vi "Vision-dynamic-pump.vi"() -> ()   [LabVIEW 2013]
doc: "Use this template to build a standard state machine design pattern. Each state executes code and determines which state to transition to. Contrast this design pattern with the User Interface Event Handler pattern, in which code executes in response to user actions. Contrast this design pattern also with the Queued Message Handler pattern, in which each message handling code can queue zero or more new messages."
uses:
  StateMachineStates 1.ctl
  <vilib>/DAQmx/read.llb/DAQmx Read (Counter DBL 1Chan 1Samp).vi
  <vilib>/DAQmx/create/channels.llb/DAQmx Create Channel (CI-Pulse Width).vi
  <vilib>/DAQmx/miscellaneous.llb/DAQmx Fill In Error Info.vi
panel:
  in  "Entrainment":bool=TRUE
  in  "Sound at \nstimulus end":bool
  in  "Manual \nvoltage (V)":dbl=2.6 format="%.2p"
  in  "Manual \nphoton #":i64=100
  out "L/R WP target":dbl
  out "List of axes":i32[](array[numeric])
  out "List of WP errors":bool[](array[boolean])
  out "WP error":bool
  out "appended array":dbl[][](array[numeric])
  out "Pump WP":dbl format="%.2f"
  in  "Trigger rate at \n52.6 degrees":dbl=2646.0 format="%.2p"
  in  "Target trial \nlength (ms)":dbl=500.0 format="%.2p"
  in  "Default pump \nWP angle":dbl=52.6
  in  "Pump WP":bool=TRUE
  out "Photon time (ms)":dbl format="%.2f"
  in  "Interval (ms)":u32
  out "Repetition":dbl
  in  "Repetitions":dbl=1.0
  out "WP time (ms)":u32
  out "VISA Handle out":refnum<visa-resource-name>="ASRL5::INSTR"
  out "Initializing":bool
  out "Trial mode":enum16{"Single Photons", "LED", "Mixed LED"}(ring)
  in  "Frequency of LED trials\nfor Mixed mode":dbl=30.0
  out "Bright trial\nrequested":bool
  out "Observer Ready":bool
  in  "Bright/mixed mode \nLED voltage (V)":dbl=2.6 min=-3.0 max=4.0 format="%.2f"
  in  "GPIB address":string="15"
  in  "Period (ms)":i64=20
  in  "Pulse \nlength (ms)":dbl=50.0
  out "L/R WP":dbl format="%.2f"
  in  "Manually \ninitialize":bool
  in  "COM for WPs":u8=3
  out "Blocked trial #":i32
  out "Photon #":i32
  out "LED Voltage":dbl
  in  "Blocking requirements":cluster{"Value":dbl, " Number":i32}[](array[cluster])
  in  "Manual":bool
  in  "Path":path=path "C:/Users/Lab/Dropbox/Vision software/Data"
  out "Counts 2":u32
  out "Counts 1":u32
  in  "Delay for APDs (ms)":u32=25
  in  "Counter 2":tag="Dev1/ctr1"
  in  "Counter 1":tag="Dev1/ctr0"
  out "Trial #":i32
  in  "Mode":enum16{"Single Photons", "LED", "Mixed"}(ring)=enum."Mixed"
  in  "Audio":bool=TRUE
  in  "Self-paced":bool
  out "Stimulus":bool
  out "Location Set":bool
  out "Stimulus \nlocation":string
  out "Waiting":bool
  out "Observer Responded":bool
  out "Response \ntime (ms)":dbl
  out "Observer \nchoice":string
  out "Confidence":i32
  in  "stop":bool
  in  "Next Trial":bool
  in  "Create New File":bool
  out "Subject #":string
  # "Settings for Blocking\nand Mixed Mode"
  # "Instructions: Run VI. Enter blocking requirements, then press\nCreate New File. Initialize waveplates if necessary, and set\nhighlighted controls to desired values. Press Next Trial to begin."
  # "Researcher Interface"
  # "Trial Options"
  # "Counter Options"
  # "Trial Information"
  # "(1)"
  # "(3)"
  # "LED Options"
  # "Pump Settings"
  # "Troubleshooting"
  # "Waveplates"
  # "(2)"
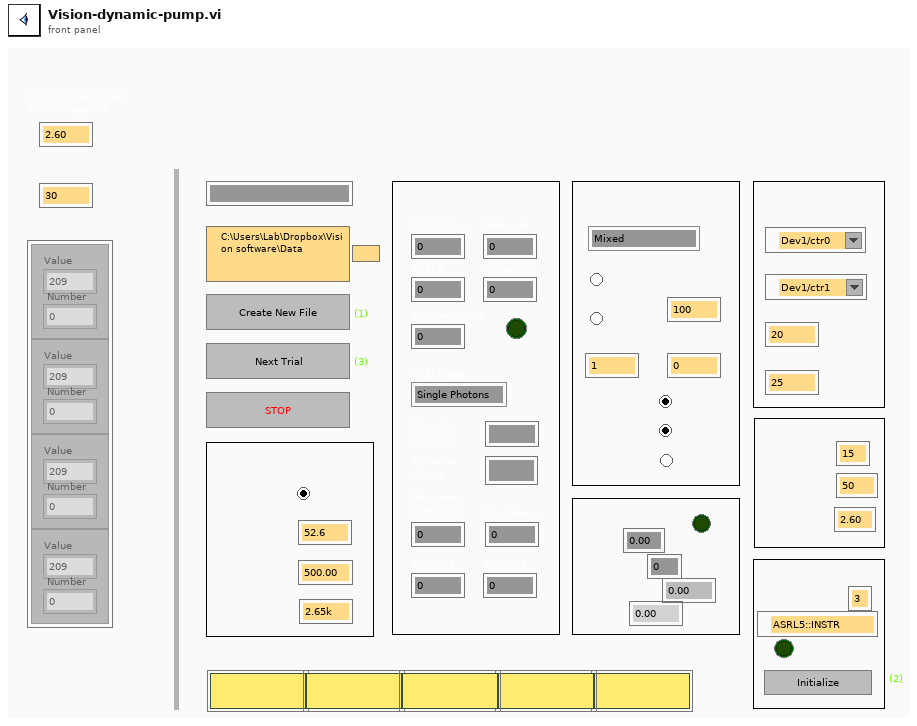
[diagram p1: front panel]
types:
  T1 = typedef "StateMachineStates 1.ctl" = enum16{"WaitResearcher", "Setup", "SetWP", "WaveplateError", "WaitObserverReady", "Photons", "LED", "WaitObserverResponse", "CleanUp", "Stop"}
  T2 = enum16{"0", "1", "2", "3", "4", "5", "6", "7", "8", "9", "A", "B", "C", "D", "E", "F", "G", "H", "I", "J", "K", "L", "M", "N", "O", "P", "Q", "R", "S", "T", "U", "V", "W", "X", "Y", "Z", "F1", "F2", "F3", "F4", "F5", "F6", "F7", "F8", "F9", "F10", "F11", "F12", "F13", "F14", "F15", "ADD", "BACK", "BACKSLASH", "CAPITAL", "COMMA", "DECIMAL", "DELETE", "DIVIDE", "DOWN", "END", "EQUALS", "ESCAPE", "GRAVE (`)", "HOME", "INSERT", "LBRACKET", "LCONTROL", "LEFT", "L ALT", "LSHIFT", "LWIN", "MINUS", "MULTIPLY", "NEXT", "NUMLOCK", "NUMPAD_0", "NUMPAD_1", "NUMPAD_2", "NUMPAD_3", "NUMPAD_4", "NUMPAD_5", "NUMPAD_6", "NUMPAD_7", "NUMPAD_8", "NUMPAD_9", "PAUSE", "PERIOD", "PRIOR (PG UP)", "RBRACKET", "RCONTROL", "RETURN", "RIGHT", "R ALT", "RSHIFT", "RWIN", "SCROLL", "SEMICOLON", "SLASH", "SPACE", "SUBTRACT", "TAB", "UP", "ENTER (num pad)", "' (quote)"}
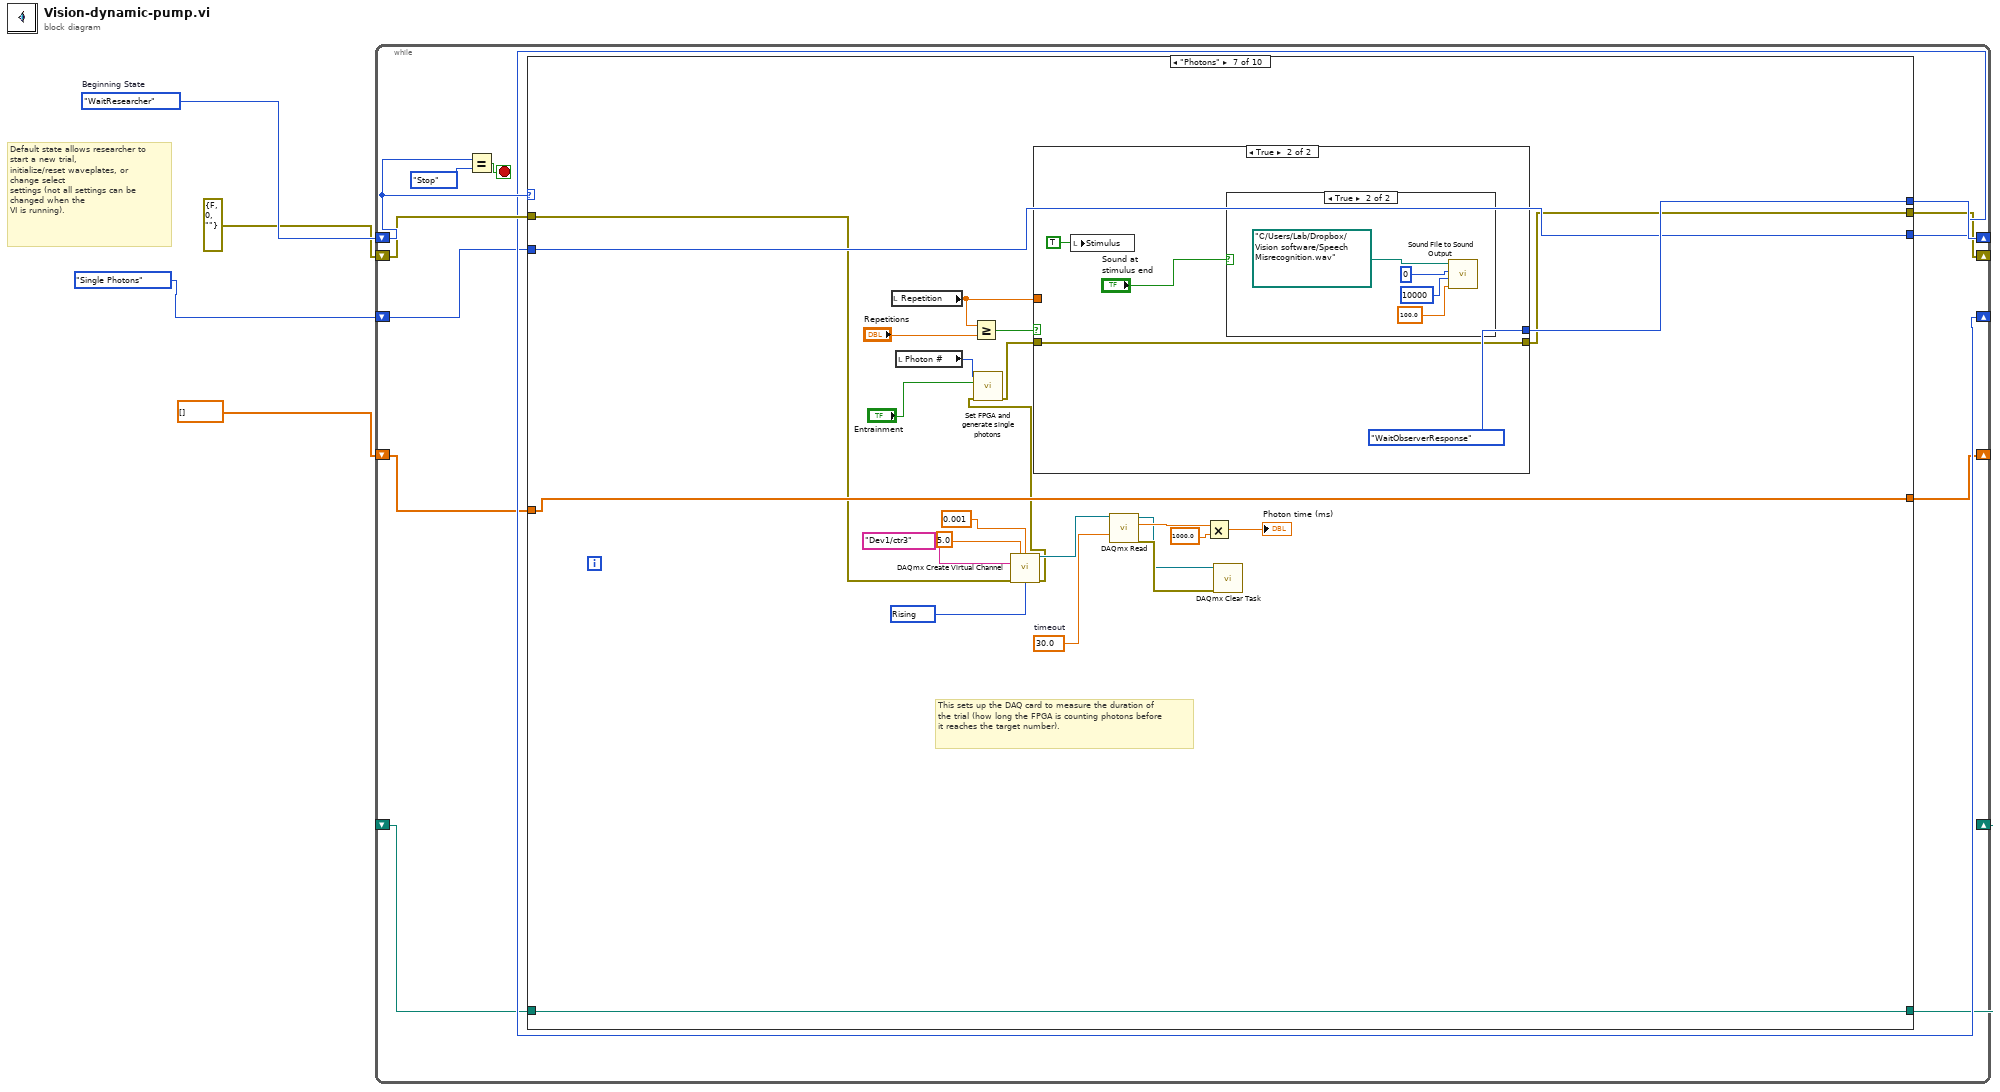
[diagram p0: block diagram]
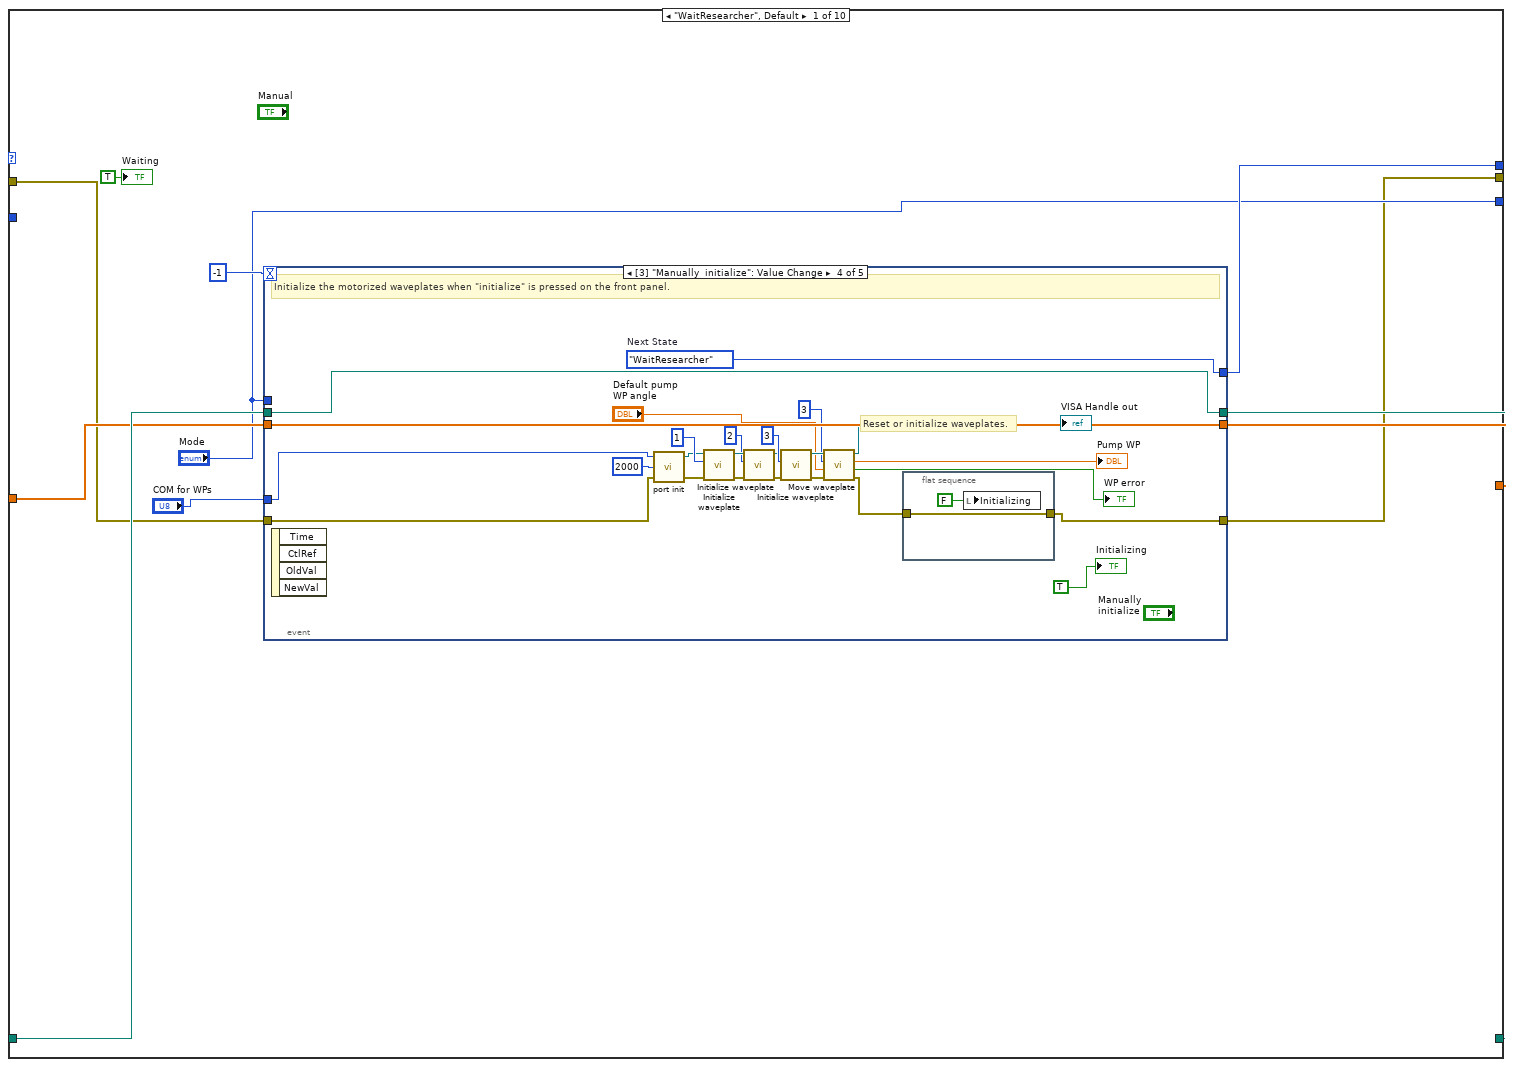
[diagram p2: hidden frame]
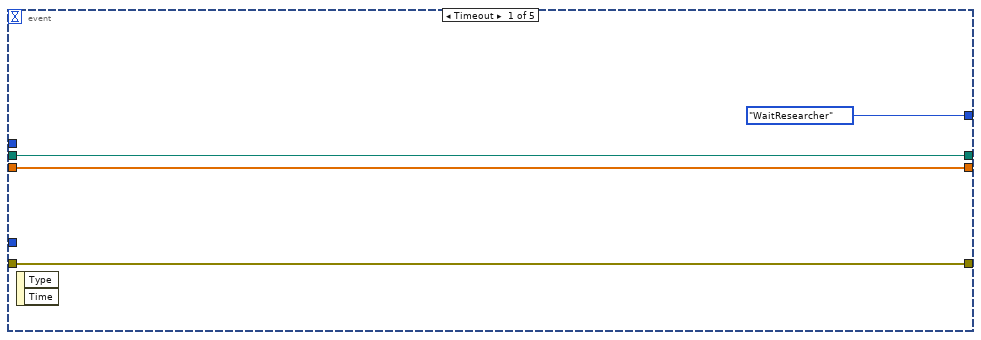
[diagram p3: hidden frame]
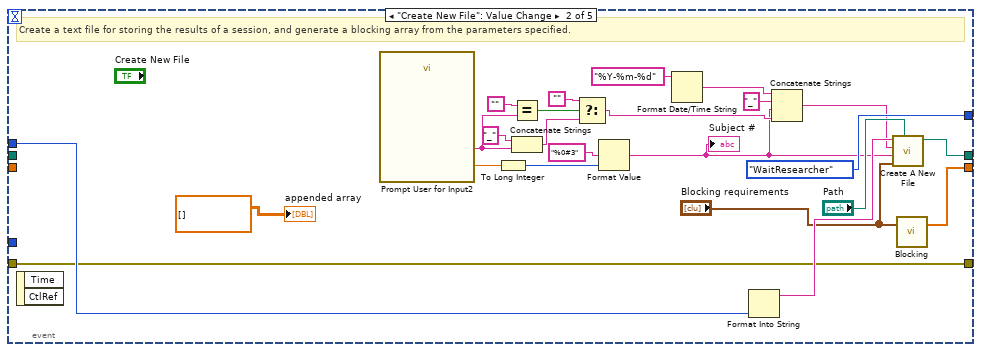
[diagram p4: hidden frame]
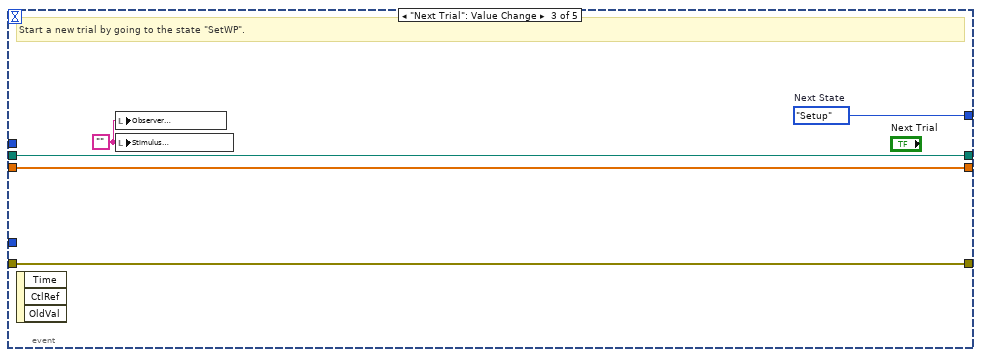
[diagram p5: hidden frame]
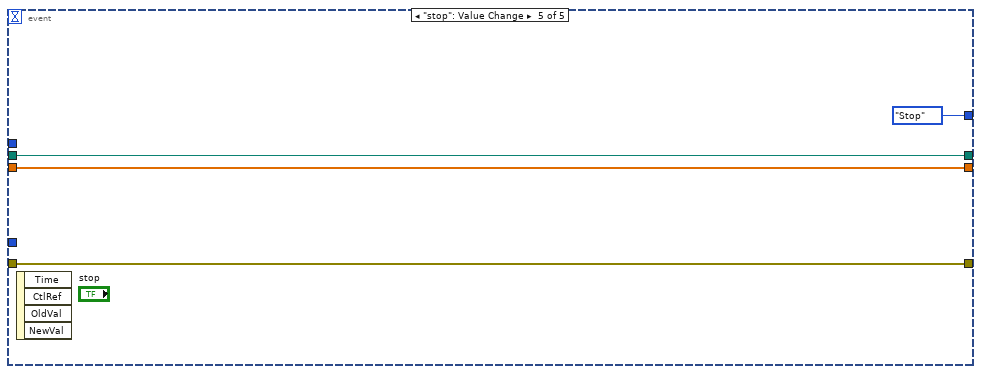
[diagram p6: hidden frame]
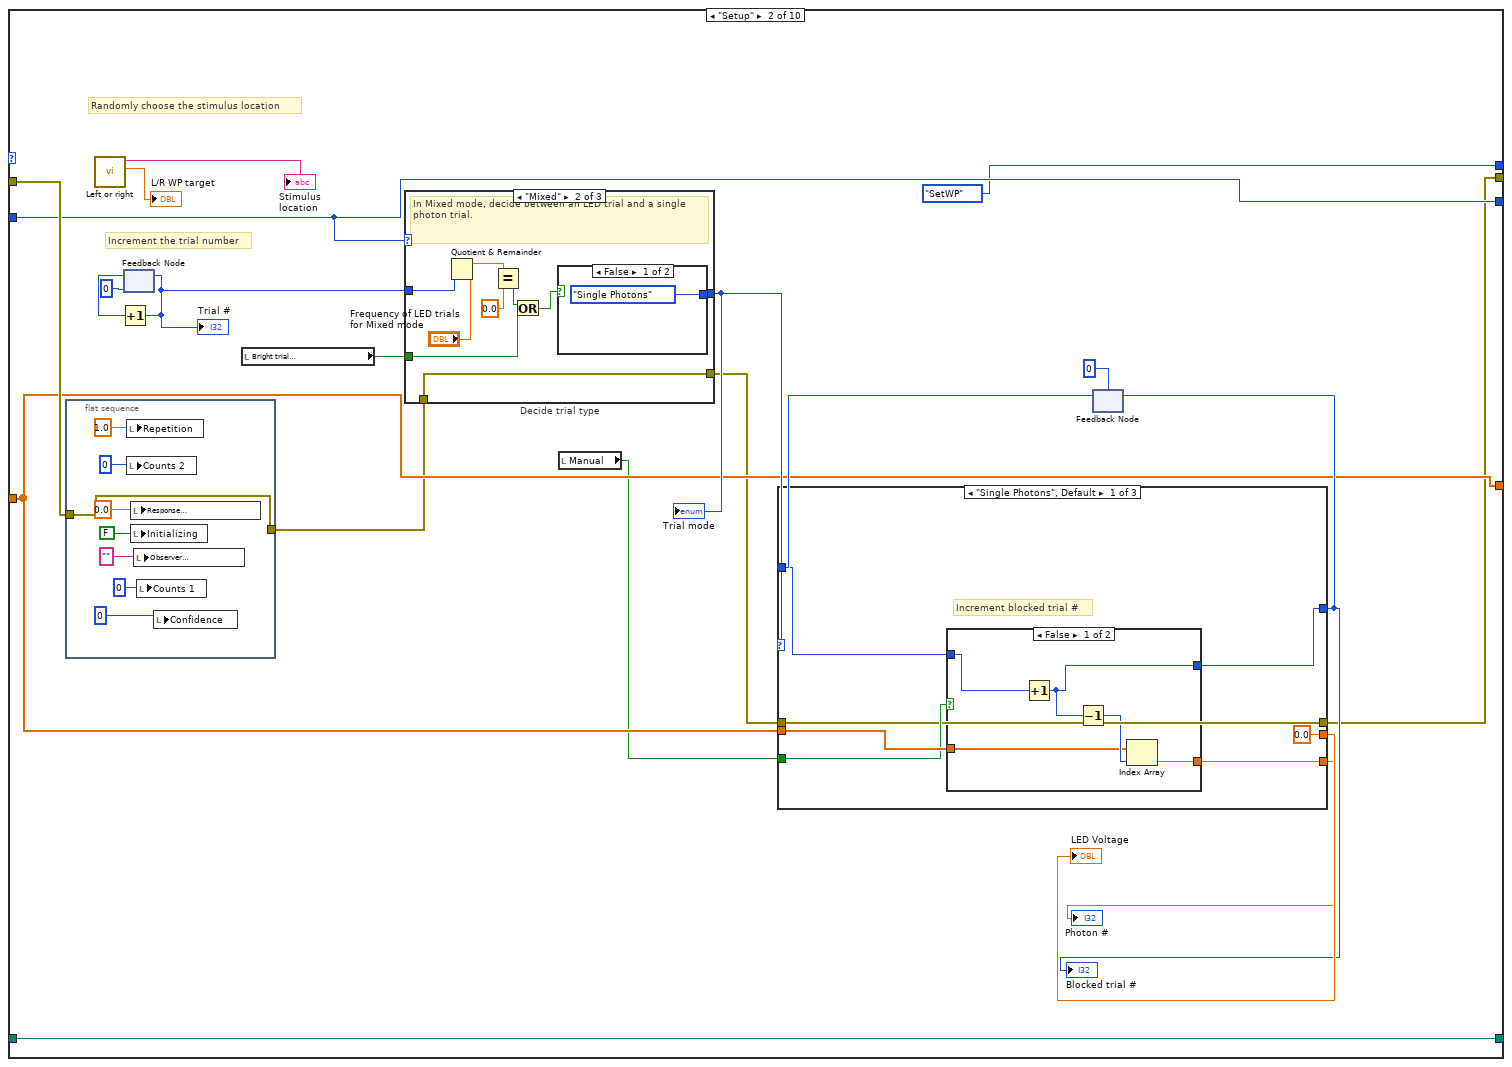
[diagram p7: hidden frame]
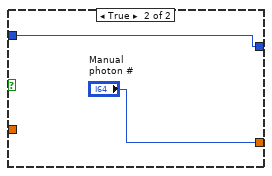
[diagram p8: hidden frame]
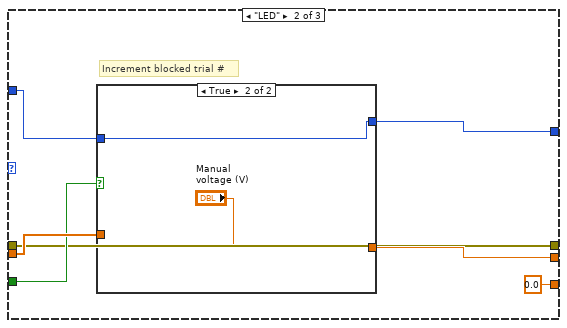
[diagram p9: hidden frame]
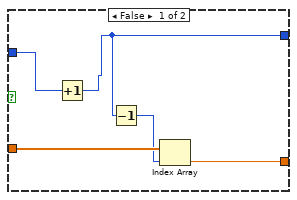
[diagram p10: hidden frame]
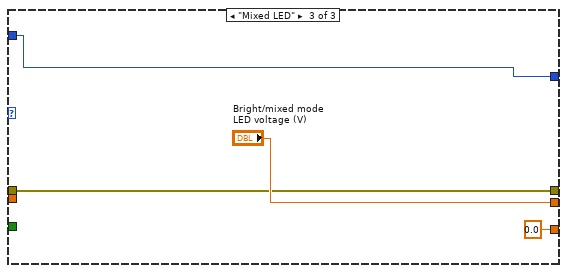
[diagram p11: hidden frame]
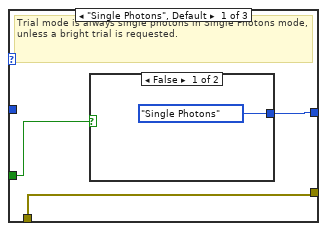
[diagram p12: hidden frame]
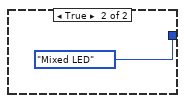
[diagram p13: hidden frame]
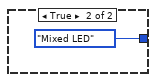
[diagram p14: hidden frame]
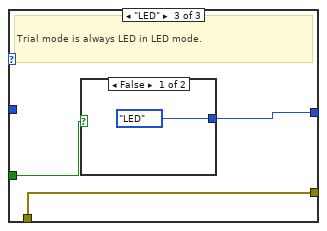
[diagram p15: hidden frame]
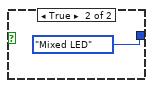
[diagram p16: hidden frame]
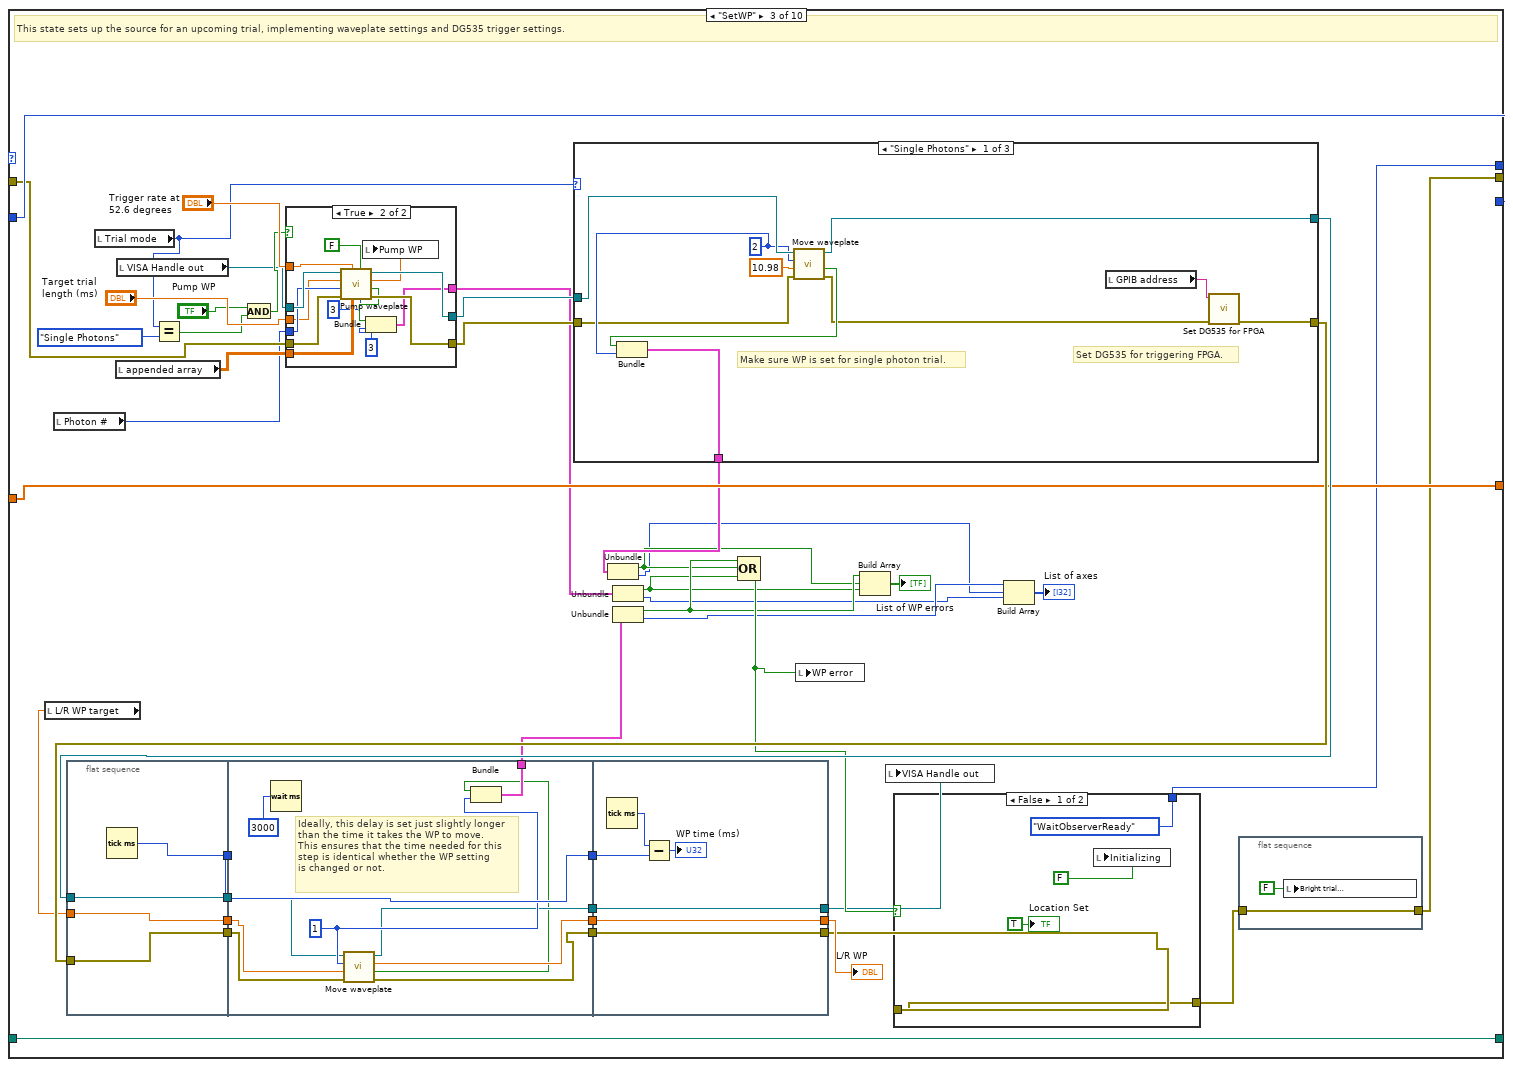
[diagram p17: hidden frame]
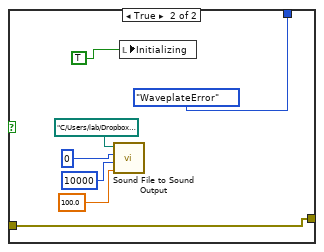
[diagram p18: hidden frame]
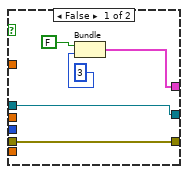
[diagram p19: hidden frame]
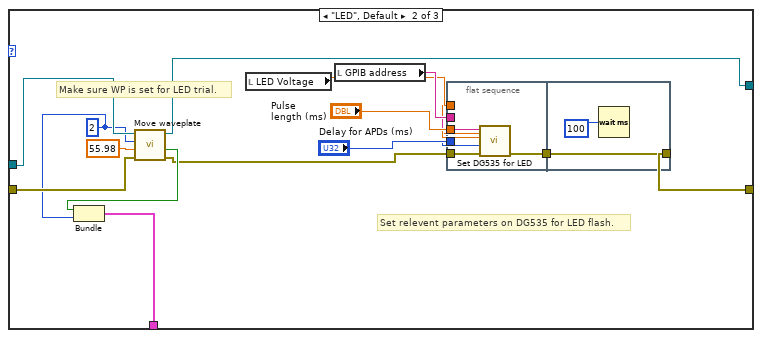
[diagram p20: hidden frame]
diagram:
  w4 = StateMachineStates_1."WaitResearcher"  # Beginning State
  # "Default state allows researcher to start a new trial,\ninitialize/reset waveplates, or change select\nsettings (not all settings can be changed when the\nVI is running)."
  n1 = while {
    shift-right: [w13] -> _
    shift-left: w4 -> [w14]
    shift-right: [w6] -> _
    shift-left: errorcluster {"status"=FALSE, "code"=0, "source"=""} ("error out") -> [w12]
    shift-right: [w11] -> _
    shift-left: enum16{"Single Photons", "LED", "Mixed"}."Single Photons" ("Mode") -> [w10]
    shift-right: [w9] -> _
    shift-left: _ -> [w5]
    shift-right: [w8] -> _
    shift-left: dbl[] [] ("Blocking array") -> [w7]
    stop <- w16 stop-if-true
    n2 = Equal?(x=w14, y=StateMachineStates_1."Stop" ("States")) -> (x = y?=w16:bool)
    n3 = case shown="\"Photons\"" w14 {
      selector: w14 -> [_ _ _ _ w383 _ _ _ _ _]
      tunnel: [w27 StateMachineStates_1."SetWP" ("Next State") w196 w332 w384 StateMachineStates_1."WaitObserverResponse" ("Next State") w454 w475 w528 w566] -> w13
      tunnel: [w18 w93 w176 w329 w376 w427 w450 w468 w519 w570] -> w6
      tunnel: w12 -> [w19 w111 w204 w333 w377 w416 w432 w469 w518 w569]
      tunnel: ["Mode" w99 w216 w336 w381 w423 w453 w474 w526 w573] -> w11
      tunnel: w10 -> [_ w99 w216 w336 w380 w423 w453 w474 w526 w573]
      tunnel: [w24 w92 w217 w334 w379 w420 w452 w473 w525 w572] -> w9
      tunnel: w5 -> [w23 w92 w217 w334 w379 w420 w452 w473 w525 w572]
      tunnel: [w22 w98 w207 w335 w378 w419 w451 w472 w523 w571] -> w8
      tunnel: w7 -> [w21 w98 w207 w335 w378 w419 w451 w472 w523 w571]
      frame "WaitResearcher", Default {
        n4 = event shown="[3] \"Manually  initialize\": Value Change" {
          selector: _ -> [_ _ _ _ _]
          dyn-events: _ -> [_ _ _ _ _]
          timeout: -1 -> [_ _ _ _ _]
          tunnel: [StateMachineStates_1."WaitResearcher" ("Next State") StateMachineStates_1."WaitResearcher" ("Next State") w56 w85 StateMachineStates_1."Stop" ("Next State")] -> w27
          tunnel: "Mode" -> [_ w51 _ _ _]
          tunnel: [w31 w45 w59 w84 w90] -> w24
          tunnel: w23 -> [w31 _ w59 w84 w90]
          tunnel: [w30 w49 w58 w82 w89] -> w22
          tunnel: w21 -> [w30 _ w58 w82 w89]
          tunnel: w19 -> [w29 w44 w57 w77 w88]
          tunnel: [w29 w44 w57 w81 w88] -> w18
          tunnel: "COM for WPs" -> [_ _ _ w78 _]
          event Timeout {
            n5 = event-data() -> ()  [unwired: 1 in, 2 out]
          }
          event "Create New File": Value Change {
            # "Create a text file for storing the results of a session, and generate a blocking array from the parameters specified."
            n6 = event-data() -> ()  [unwired: 1 in, 2 out]
            n7 = call "Prompt User for Input2"() -> ("Subject #"=w54:dbl, "Filename"=w39:string)  [unwired: 16 in, 2 out]
            n8 = To Long Integer(number=w54) -> (32bit integer=w35:i32)
            n9 = Equal?(x="", y=w39) -> (x = y?=w52:bool)
            n10 = Concatenate Strings("_" ("string"), w39) -> (w42:string)
            n11 = Select(t="", s=w52, f=w42) -> (s? t:f=w37:string)
            n12 = Format Value(format string="%0#3", value (0)=w35) -> (output string=w34:string)  [unwired: 1 in]
            "Subject #" <- w34
            n13 = Format Date/Time String(time format string (%c)="%Y-%m-%d") -> (date/time string=w40:string)  [unwired: 2 in]
            n14 = Format Into String(w51) -> (resulting string=w50:string)  [unwired: 3 in, 1 out]
            n15 = Concatenate Strings(w40, "_" ("string"), w34, w37) -> (w46:string)
            n16 = call "Create A New File.vi"("Path in"="Path", "Blocking requirements"="Blocking requirements", "Subject #"=w34, "Filename"=w46, "Mode"=w50) -> ("Path out"=w45:path)  [unwired: 6 in]
            n17 = call "Blocking.vi"("Blocking requirements"="Blocking requirements") -> ("Blocking array"=w49:dbl[])  [unwired: 2 in]
            "appended array" <- dbl[][] []
          }
          event "Next Trial": Value Change {
            w56 = StateMachineStates_1."Setup"  # Next State
            w60 = ""
            # "Start a new trial by going to the state \"SetWP\"."
            n18 = event-data() -> ()  [unwired: 1 in, 3 out]
            n19 = local write "Observer \nchoice"(w60) -> ()
            n20 = local write "Stimulus \nlocation"(w60) -> ()
          }
          event "Manually \ninitialize": Value Change {
            w85 = StateMachineStates_1."WaitResearcher"  # Next State
            # "Reset or initialize waveplates."
            # "Initialize the motorized waveplates when \"initialize\" is pressed on the front panel."
            n21 = event-data() -> ()  [unwired: 1 in, 4 out]
            n22 = call "port init.vi"("error in"=w77, "Timeout (ms)"=u32 2000 ("Timeout (300 ms)"), "SerialPort"=w78) -> ("error out"=w76:errorcluster, "Visa Handle"=w75:refnum<visa-resource-name>)  [unwired: 1 in]
            n23 = call "Initialize waveplate.vi"("error in (no error)"=w76, "Axis in"=1, "VISA Handle in"=w75) -> ("error out"=w72:errorcluster, "VISA Refnum out"=w74:refnum<visa-resource-name>)  [unwired: 6 in, 1 out]
            n24 = call "Initialize waveplate.vi"("error in (no error)"=w72, "Axis in"=2, "VISA Handle in"=w74) -> ("error out"=w69:errorcluster, "VISA Refnum out"=w70:refnum<visa-resource-name>)  [unwired: 6 in, 1 out]
            n25 = call "Initialize waveplate.vi"("error in (no error)"=w69, "Axis in"=3, "VISA Handle in"=w70) -> ("error out"=w65:errorcluster, "VISA Refnum out"=w68:refnum<visa-resource-name>)  [unwired: 6 in, 1 out]
            n26 = call "Move waveplate.vi"("error in (no error)"=w65, "Angle"="Default pump \nWP angle", "Axis in"=3, "VISA Refnum in"=w68) -> ("error out"=w64:errorcluster, "WP Error"=→"WP error":bool, "Current position (units)"=→"Pump WP":dbl, "VISA Refnum out"=→"VISA Handle out":refnum<visa-resource-name>)  [unwired: 4 in]
            n27 = flat-sequence {
              tunnel: w64 -> [w87]
              tunnel: [w87] -> w81
              frame #0 {
                n28 = local write "Initializing"(FALSE ("Initializing waveplates")) -> ()
              }
            }
            "Initializing" <- TRUE ("Initializing waveplates")
          }
          event "stop": Value Change {
            n29 = event-data() -> ()  [unwired: 1 in, 4 out]
          }
        }
        "Waiting" <- TRUE ("Waiting")
      }
      frame "Setup" {
        # "Randomly choose the stimulus location"
        # "Increment the trial number"
        n30 = flat-sequence {
          tunnel: w111 -> [w145]
          tunnel: [w145] -> w95
          frame #0 {
            n31 = local write "Repetition"(1.0 ("Repitition #")) -> ()
            n32 = local write "Counts 2"(u32 0 ("Counts 2")) -> ()
            n33 = local write "Response \ntime (ms)"(0.0 ("Response \ntime (ms)")) -> ()
            n34 = local write "Initializing"(FALSE ("Initializing waveplates")) -> ()
            n35 = local write "Observer \nchoice"("" ("Observer \nchoice")) -> ()
            n36 = local write "Counts 1"(u32 0 ("Counts 1")) -> ()
            n37 = local write "Confidence"(0 ("Confidence")) -> ()
          }
        }
        n38 = call "Left or right.vi"() -> ("New target position (units)"=→"L/R WP target":dbl, "String"=→"Stimulus \nlocation":string)  [unwired: 10 in]
        n39 = feedback #1(0 ("x+1")) -> (w110:i32)
        n40 = Increment(x=w110) -> (x+1=w108:i32)
        "Trial #" <- w108
        n41 = feedback-in #1(w108) -> ()
        n42 = local read "Bright trial\nrequested"() -> (w100:bool)
        n43 = case "Decide trial type" shown="\"Mixed\"" w99 {
          tunnel: [w155 w165 w171] -> w107
          tunnel: w108 -> [_ w166 _]
          tunnel: w100 -> [w154 w159 w170]
          tunnel: w95 -> [w153 w158 w169]
          tunnel: [w153 w158 w169] -> w94
          frame "Single Photons", Default {
            # "Trial mode is always single photons in Single Photons mode, unless a bright trial is requested."
            n44 = case shown="False" w154 {
              tunnel: [enum16{"Single Photons", "LED", "Mixed LED"}."Single Photons" ("Mode") enum16{"Single Photons", "LED", "Mixed LED"}."Mixed LED" ("Mode")] -> w155
              frame False {
              }
              frame True {
              }
            }
          }
          frame "Mixed" {
            # "In Mixed mode, decide between an LED trial and a single photon trial."
            n45 = Quotient & Remainder(x=w166, y="Frequency of LED trials\nfor Mixed mode") -> (x-y*floor(x/y)=w163:dbl)  [unwired: 1 out]
            n46 = Equal?(x=w163, y=0.0) -> (x = y?=w161:bool)
            n47 = Or(x=w161, y=w159) -> (x .or. y?=w160:bool)
            n48 = case shown="False" w160 {
              tunnel: [enum16{"Single Photons", "LED", "Mixed LED"}."Single Photons" ("Mode") enum16{"Single Photons", "LED", "Mixed LED"}."Mixed LED" ("Mode")] -> w165
              frame False {
              }
              frame True {
              }
            }
          }
          frame "LED" {
            # "Trial mode is always LED in LED mode."
            n49 = case shown="False" w170 {
              tunnel: [enum16{"Single Photons", "LED", "Mixed LED"}."LED" ("Mode") enum16{"Single Photons", "LED", "Mixed LED"}."Mixed LED" ("Mode")] -> w171
              frame False {
              }
              frame True {
              }
            }
          }
        }
        "Trial mode" <- w107
        n50 = local read "Manual"() -> (w97:bool)
        n51 = feedback #2(0 ("x+1")) -> (w103:i32)
        n52 = case shown="\"Single Photons\", Default" w107 {
          tunnel: [w116 w132 w142] -> w102
          tunnel: w98 -> [w119 w133 _]
          tunnel: [0.0 ("Value") w131 "Bright/mixed mode \nLED voltage (V)"] -> w106
          tunnel: [w118 0.0 ("Value") 0.0 ("Value")] -> w105
          tunnel: w103 -> [w115 w129 w142]
          tunnel: w97 -> [w114 w128 _]
          tunnel: w94 -> [w113 w127 w141]
          tunnel: [w113 w127 w141] -> w93
          frame "Single Photons", Default {
            # "Increment blocked trial #"
            n53 = case shown="False" w114 {
              tunnel: w119 -> [w123 _]
              tunnel: [w122 "Manual \nphoton #"] -> w118
              tunnel: [w121 w125] -> w116
              tunnel: w115 -> [w120 w125]
              frame False {
                n54 = Increment(x=w120) -> (x+1=w121:i32)
                n55 = Decrement(x=w121) -> (x-1=w124:i32)
                n56 = Index Array(array=w123, index=w124) -> (element=w122:dbl)
              }
              frame True {
              }
            }
          }
          frame "LED" {
            # "Increment blocked trial #"
            n57 = case shown="True" w128 {
              tunnel: w133 -> [w138 _]
              tunnel: [w137 w139] -> w132
              tunnel: [w135 "Manual \nvoltage (V)"] -> w131
              tunnel: w129 -> [w134 w139]
              frame False {
                n58 = Increment(x=w134) -> (x+1=w137:i32)
                n59 = Decrement(x=w137) -> (x-1=w136:i32)
                n60 = Index Array(array=w138, index=w136) -> (element=w135:dbl)
              }
              frame True {
              }
            }
          }
          frame "Mixed LED" {
          }
        }
        "Photon #" <- w105
        "Blocked trial #" <- w102
        "LED Voltage" <- w106
        n61 = feedback-in #2(w102) -> ()
      }
      frame "SetWP" {
        # "This state sets up the source for an upcoming trial, implementing waveplate settings and DG535 trigger settings."
        n62 = local read "L/R WP target"() -> (w180:dbl)
        n63 = local read "Photon #"() -> (w181:i32)
        n64 = flat-sequence {
          tunnel: w215 -> [w253]
          tunnel: w214 -> [w254]
          tunnel: [w254] -> w213
          tunnel: [w253] -> w212
          tunnel: [w252] -> w208
          tunnel: w180 -> [w251]
          tunnel: [w251] -> w179
          tunnel: w213 -> [w262]
          tunnel: w212 -> [w259]
          tunnel: [w256] -> w211
          tunnel: [w257] -> w210
          tunnel: [w264] -> w209
          tunnel: w208 -> [w264]
          tunnel: [w263] -> w191
          tunnel: [w258] -> w182
          tunnel: w179 -> [w261]
          tunnel: [w269] -> w174
          tunnel: [w270] -> w195
          tunnel: [w271] -> w218
          tunnel: w211 -> [w270]
          tunnel: w210 -> [w269]
          tunnel: w209 -> [w268]
          tunnel: w182 -> [w271]
          frame #0 {
            n65 = Tick Count (ms)() -> (millisecond timer value=w252:u32)
          }
          frame #1 {
            w260 = 1 ("Axis in")
            # "Ideally, this delay is set just slightly longer\nthan the time it takes the WP to move.\nThis ensures that the time needed for this\nstep is identical whether the WP setting\nis changed or not."
            n66 = Wait (ms)(milliseconds to wait=u32 3000) -> ()  [unwired: 1 out]
            n67 = call "Move waveplate.vi"("error in (no error)"=w262, "Angle"=w261, "Axis in"=w260, "VISA Refnum in"=w259) -> ("error out"=w256:errorcluster, "WP Error"=w255:bool, "Current position (units)"=w258:dbl, "VISA Refnum out"=w257:refnum<visa-resource-name>)  [unwired: 4 in]
            n68 = Bundle("WP Error"=w255, "Axis in"=w260) -> (w263:cluster{"WP Error":bool, "Axis in":i32})  [unwired: 1 in]
          }
          frame #2 {
            n69 = Tick Count (ms)() -> (millisecond timer value=w267:u32)
            n70 = Subtract(x=w267, y=w268) -> (x-y=→"WP time (ms)":u32)
          }
        }
        n71 = local read "Trial mode"() -> (w178:enum16{"Single Photons", "LED", "Mixed LED"})
        n72 = local read "appended array"() -> (w201:dbl[][])
        n73 = local read "VISA Handle out"() -> (w175:refnum<visa-resource-name>)
        n74 = Equal?(x=w178, y=enum16{"Single Photons", "LED", "Mixed LED"}."Single Photons") -> (x = y?=w198:bool)
        n75 = And(x="Pump WP", y=w198) -> (x .and. y?=w197:bool)
        n76 = case shown="True" w197 {
          tunnel: w175 -> [w236 w250]
          tunnel: [w236 w249] -> w206
          tunnel: w204 -> [w235 w248]
          tunnel: [w235 w247] -> w205
          tunnel: w181 -> [_ w246]
          tunnel: "Target trial \nlength (ms)" -> [_ w245]
          tunnel: "Trigger rate at \n52.6 degrees" -> [_ w244]
          tunnel: w201 -> [_ w242]
          tunnel: [w233 w238] -> w192
          frame False {
            n77 = Bundle(FALSE, 3) -> (w233:cluster{bool, i32})  [unwired: 1 in]
          }
          frame True {
            n78 = call "Pump waveplate.vi"("Axis in"=3, "Trigger rate warnings?"=FALSE, "appended array"=w242, "Trigger rate \nat 52.6 degrees"=w244, "error in (no error)"=w248, "Photon #"=w246, "Target trial \nlength (ms)"=w245, "VISA Refnum in"=w250) -> ("error out"=w247:errorcluster, "WP Error"=w240:bool, "Current position (units)"=w243:dbl, "VISA Refnum out"=w249:refnum<visa-resource-name>)
            n79 = local write "Pump WP"(w243) -> ()
            n80 = Bundle("WP Error"=w240, 3) -> (w238:cluster{"WP Error":bool, i32})  [unwired: 1 in]
          }
        }
        n81 = case shown="\"Single Photons\"" w178 {
          tunnel: w205 -> [w274 w288 w308]
          tunnel: [w280 w291 w313] -> w214
          tunnel: w206 -> [w278 w289 w311]
          tunnel: [w272 w283 w305] -> w215
          tunnel: [w279 w290 w312] -> w193
          frame "Single Photons" {
            w276 = 2 ("Axis in")
            # "Set DG535 for triggering FPGA."
            # "Make sure WP is set for single photon trial."
            n82 = call "Move waveplate.vi"("error in (no error)"=w274, "Angle"=10.98 ("New target position (units)"), "Axis in"=w276, "VISA Refnum in"=w278) -> ("error out"=w273:errorcluster, "WP Error"=w275:bool, "VISA Refnum out"=w272:refnum<visa-resource-name>)  [unwired: 4 in, 1 out]
            n83 = Bundle("WP Error"=w275, "Axis in"=w276) -> (w279:cluster{"WP Error":bool, "Axis in":i32})  [unwired: 1 in]
            n84 = local read "GPIB address"() -> (w281:string)
            n85 = call "Set DG535 for FPGA.vi"("error in (no error)"=w273, "GPIB address"=w281) -> ("error out"=w280:errorcluster)  [unwired: 9 in]
          }
          frame "LED", Default {
            w286 = 2 ("Axis in")
            # "Make sure WP is set for LED trial."
            # "Set relevent parameters on DG535 for LED flash."
            n86 = call "Move waveplate.vi"("error in (no error)"=w288, "Angle"=55.98 ("New target position (units)"), "Axis in"=w286, "VISA Refnum in"=w289) -> ("error out"=w284:errorcluster, "WP Error"=w285:bool, "VISA Refnum out"=w283:refnum<visa-resource-name>)  [unwired: 4 in, 1 out]
            n87 = Bundle("WP Error"=w285, "Axis in"=w286) -> (w290:cluster{"WP Error":bool, "Axis in":i32})  [unwired: 1 in]
            n88 = local read "LED Voltage"() -> (w282:dbl)
            n89 = local read "GPIB address"() -> (w295:string)
            n90 = flat-sequence {
              tunnel: "Delay for APDs (ms)" -> [w301]
              tunnel: w295 -> [w300]
              tunnel: "Pulse \nlength (ms)" -> [w299]
              tunnel: w282 -> [w298]
              tunnel: w284 -> [w297]
              tunnel: [w296] -> w292
              tunnel: w292 -> [w302]
              tunnel: [w302] -> w291
              frame #0 {
                n91 = call "Set DG535 for LED.vi"("amplitude"=w298, "error in"=w297, "Delay (ms)"=w301, "Pulse length (ms)"=w299, "GPIB address"=w300) -> ("error out"=w296:errorcluster)  [unwired: 6 in]
              }
              frame #1 {
                n92 = Wait (ms)(milliseconds to wait=u32 100) -> ()  [unwired: 1 out]
              }
            }
          }
          frame "Mixed LED" {
            w310 = 2 ("Axis in")
            # "Make sure WP is set for LED trial."
            n93 = local read "Bright/mixed mode \nLED voltage (V)"() -> (w304:dbl)
            n94 = call "Move waveplate.vi"("error in (no error)"=w308, "Angle"=55.98 ("New target position (units)"), "Axis in"=w310, "VISA Refnum in"=w311) -> ("error out"=w307:errorcluster, "WP Error"=w306:bool, "VISA Refnum out"=w305:refnum<visa-resource-name>)  [unwired: 4 in, 1 out]
            n95 = Bundle("WP Error"=w306, "Axis in"=w310) -> (w312:cluster{"WP Error":bool, "Axis in":i32})  [unwired: 1 in]
            n96 = local read "Delay for APDs (ms)"() -> (w315:u32)
            n97 = local read "Pulse \nlength (ms)"() -> (w316:dbl)
            n98 = local read "GPIB address"() -> (w317:string)
            n99 = flat-sequence {
              tunnel: w315 -> [w322]
              tunnel: w317 -> [w321]
              tunnel: w316 -> [w320]
              tunnel: w304 -> [w319]
              tunnel: w307 -> [w318]
              tunnel: [w318] -> w314
              tunnel: w314 -> [w323]
              tunnel: [w323] -> w313
              frame #0 {
                n100 = call "Set DG535 for LED.vi"("amplitude"=w319, "Delay (ms)"=w322, "Pulse length (ms)"=w320, "GPIB address"=w321) -> ()  [unwired: 7 in, 1 out]
              }
              frame #1 {
                n101 = Wait (ms)(milliseconds to wait=u32 100) -> ()  [unwired: 1 out]
              }
            }
          }
        }
        n102 = Unbundle(w193) -> ("WP Error"=w189:bool, "Axis in"=w185:i32)
        n103 = Unbundle(w192) -> ("WP Error"=w188:bool, w184:i32)
        n104 = Unbundle(w191) -> ("WP Error"=w190:bool, "Axis in"=w186:i32)
        n105 = Compound Arithmetic op=OR(w190, w189, w188) -> (w194:bool)
        n106 = local write "WP error"(w194) -> ()
        n107 = Build Array(w190, w189, w188) -> (→"List of WP errors":bool[])
        n108 = local write "VISA Handle out"(w174) -> ()
        n109 = case shown="False" w194 {
          tunnel: [StateMachineStates_1."WaitObserverReady" ("Next State") StateMachineStates_1."WaveplateError" ("Next State")] -> w196
          tunnel: w195 -> [w221 w229]
          tunnel: [w221 w229] -> w177
          frame False {
            n110 = local write "Initializing"(FALSE ("WP Error")) -> ()
            "Location Set" <- TRUE ("Location Set")
          }
          frame True {
            n111 = call "Sound File to Sound Output.vi"("Volume"=100.0, "Number of Samples/Iteration"=10000, "Device ID"=u32 0, "File Path"=path "C:/Users/lab/Dropbox/Vision software/Source/Windows Critical Stop.wav") -> ()
            n112 = local write "Initializing"(TRUE ("WP Error")) -> ()
          }
        }
        n113 = Build Array(w186, w185, w184) -> (→"List of axes":i32[])
        n114 = flat-sequence {
          tunnel: w177 -> [w220]
          tunnel: [w220] -> w176
          frame #0 {
            n115 = local write "Bright trial\nrequested"(FALSE ("Bright trial\nrequested")) -> ()
          }
        }
        "L/R WP" <- w218
      }
      frame "WaveplateError" {
        n116 = local read "VISA Handle out"() -> (w325:refnum<visa-resource-name>)
        n117 = call <vilib>:"Clear Errors.vi"("error in (no error)"=w333) -> ("error out"=w330:errorcluster)  [unwired: 6 in]
        n118 = local read "List of WP errors"() -> (w331:bool[])
        n119 = for {
          tunnel: w331 -> [w347] mode=indexing
          tunnel: w330 -> [w343]
          tunnel: [w342] -> w329
          tunnel: [w340] -> w327 mode=indexing
          shift-right: [w341] -> w328
          shift-left: w325 -> [w339]
          i -> [w345]
          n120 = local read "List of axes"() -> (w346:i32[])
          n121 = Index Array(array=w346, index=w345) -> (element=w344:i32)
          n122 = case shown="True" w347 {
            tunnel: w344 -> [_ w363]
            tunnel: w343 -> [w350 w364]
            tunnel: [w350 w360] -> w342
            tunnel: w339 -> [w349 w359]
            tunnel: [w349 w357] -> w341
            tunnel: [FALSE ("WP Error") w352] -> w340
            frame False {
            }
            frame True {
              n123 = local read "Pump WP"() -> (w354:bool)
              n124 = Not(x=w354) -> (.not. x?=w353:bool)
              n125 = call "Initialize waveplate.vi"("error in (no error)"=w364, "Axis in"=w363, "VISA Handle in"=w359) -> ("error out"=w361:errorcluster, "WP Error"=w351:bool, "VISA Refnum out"=w358:refnum<visa-resource-name>)  [unwired: 6 in]
              n126 = Equal?(x=3, y=w363) -> (x = y?=w356:bool)
              n127 = And(x=w353, y=w356) -> (x .and. y?=w355:bool)
              n128 = case shown="True" w355 {
                tunnel: w361 -> [w367 w372]
                tunnel: [w367 w371] -> w360
                tunnel: w358 -> [w366 w370]
                tunnel: [w366 w369] -> w357
                tunnel: [w365 w368] -> w352
                tunnel: w351 -> [w365 _]
                frame False {
                }
                frame True {
                  n129 = local read "Default pump \nWP angle"() -> (w374:dbl)
                  n130 = call "Move waveplate.vi"("error in (no error)"=w372, "Angle"=w374, "Axis in"=3, "VISA Refnum in"=w370) -> ("error out"=w371:errorcluster, "WP Error"=w368:bool, "Current position (units)"=w375:dbl, "VISA Refnum out"=w369:refnum<visa-resource-name>)  [unwired: 4 in]
                  n131 = local write "Pump WP"(w375) -> ()
                }
              }
            }
          }
        }
        n132 = local write "VISA Handle out"(w328) -> ()
        n133 = Or Array Elements(Boolean array=w327) -> (logical OR=w326:bool)
        n134 = case shown="True" w326 {
          tunnel: [StateMachineStates_1."SetWP" ("Next State") StateMachineStates_1."WaveplateError" ("Next State")] -> w332
          frame False {
          }
          frame True {
          }
        }
      }
      frame "WaitObserverReady" {
        # "Wait for the observer to trigger the beginning of a trial by pressing the spacebar, then go to a stimulus-producing state determined by \"mode\" on the front panel."
        n135 = flat-sequence {
          tunnel: [w386] -> w382
          tunnel: w377 -> [w386]
          tunnel: w383 -> [w397]
          tunnel: w382 -> [w395]
          tunnel: w380 -> [w390]
          tunnel: [w391] -> w376
          tunnel: [w398] -> w384
          tunnel: [w394] -> w381
          frame #0 {
            n136 = local read "Bright/mixed mode \nLED voltage (V)"() -> (w385:dbl)
            n137 = local read "LED Voltage"() -> (w387:dbl)
            n138 = call "Play sound start trial.vi"("LED Voltage"=w387, "Bright/mixed mode \nLED voltage (V)"=w385) -> ()  [unwired: 10 in]
          }
          frame #1 {
            n139 = local read "Trial mode"() -> (w389:enum16{"Single Photons", "LED", "Mixed LED"})
            n140 = call "Query Keyboard.vi"("error in (no error)"=w395, "Stop?"=FALSE) -> ("error out"=w392:errorcluster, "element"=w396:T2)  [unwired: 8 in]
            n141 = case shown="\"NUMPAD_0\"" w396 {
              tunnel: [StateMachineStates_1."WaitObserverReady" ("Next State") w407 StateMachineStates_1."WaitObserverReady" ("Next State")] -> w398
              tunnel: w397 -> [_ _ _]
              tunnel: [w401 w406 w414] -> w394
              tunnel: w390 -> [w401 w406 w414]
              tunnel: w392 -> [w400 w405 w411]
              tunnel: [w400 w405 w411] -> w391
              tunnel: w389 -> [_ w404 _]
              tunnel: [FALSE ("Observer Ready") TRUE ("Observer Ready") FALSE ("Observer Ready")] -> w388
              frame "1", Default {
              }
              frame "SPACE" {
                # "If the subject presses SPACE, move to the appropriate stimulus-producing mode (either Photons, Detectors, or LED)."
                n142 = case shown="\"Single Photons\", Default" w404 {
                  tunnel: [w408 w409 w410] -> w407
                  frame "Single Photons", Default {
                    w408 = StateMachineStates_1."Photons"  # Next State
                  }
                  frame "LED" {
                    w409 = StateMachineStates_1."LED"  # Next State
                  }
                  frame "Mixed LED" {
                    w410 = StateMachineStates_1."LED"  # Next State
                  }
                }
              }
              frame "NUMPAD_0" {
                # "If the subject presses 0, set the \"bright trial requested\" flag and keep waiting for a response"
                "Bright trial\nrequested" <- TRUE ("Bright trial\nrequested")
              }
            }
            "Observer Ready" <- w388
          }
        }
      }
      frame "LED" {
        # "Flash LED while reading out counts from two single-photon detectors."
        n143 = call "flashLED_DG535andcount.vi"("error in"=w416, "GPIB address"="GPIB address", "Period"="Period (ms)", "Counter 2"="Counter 2", "Counter 1"="Counter 1") -> ("Counts 2"=→"Counts 2":u32, "Counts 1"=→"Counts 1":u32, "error out"=w426:errorcluster)  [unwired: 4 in]
        n144 = flat-sequence {
          tunnel: w426 -> [w429]
          tunnel: [w429] -> w427
          frame #0 {
            "Stimulus" <- TRUE ("Stimulus")
          }
        }
      }
      frame "Photons" {
        w442 = 30.0  # timeout
        w439 = 10280 items=["Rising"=10280, "Falling"=10171] ("Starting Edge")
        # "This sets up the DAQ card to measure the duration of the trial (how long the FPGA is counting photons before it reaches the target number)."
        n145 = local read "Repetition"() -> (w447:dbl)
        n146 = local read "Photon #"() -> (w445:i32)
        n147 = Greater Or Equal?(x=w447, y="Repetitions") -> (x >= y?=w449:bool)
        n148 = call-poly <vilib>:"DAQmx Create Virtual Channel.vi"("maximum value"=5.0 ("Maximum Value (sec)"), "minimum value"=0.001 ("Minimum Value (sec)"), "counter"=tag "Dev1/ctr3" ("Physical Channel"), "error in"=w432, "starting edge"=w439) -> ("task out"=w438:refnum<k21>, "error out"=w433:errorcluster)  [unwired: 9 in]
        n149 = call "Set FPGA and generate single photons.vi"("error in (no error)"=w433, "Entrainment"="Entrainment", "Photon #"=w445) -> ("error out"=w446:errorcluster)  [unwired: 8 in]
        n150 = case shown="True" w449 {
          tunnel: [StateMachineStates_1."Photons" ("States") StateMachineStates_1."WaitObserverResponse" ("States")] -> w454
          tunnel: w446 -> [w458 w462]
          tunnel: [w458 w462] -> w450
          tunnel: w447 -> [w457 _]
          frame False {
            n151 = Wait (ms)(milliseconds to wait="Interval (ms)") -> ()  [unwired: 1 out]
            n152 = Increment(x=w457) -> (x+1=→"Repetition":dbl)
          }
          frame True {
            n153 = local write "Stimulus"(TRUE ("Counts Taken")) -> ()
            n154 = case shown="True" "Sound at \nstimulus end" {
              frame False {
              }
              frame True {
                n155 = call "Sound File to Sound Output.vi"("Volume"=100.0, "Number of Samples/Iteration"=10000, "Device ID"=u32 0, "File Path"=path "C:/Users/Lab/Dropbox/Vision software/Speech Misrecognition.wav") -> ()
              }
            }
          }
        }
        n156 = call-poly <vilib>:"DAQmx Read.vi"("task/channels in"=w438, "timeout"=w442) -> ("task out"=w440:refnum<k21>, "data"=w444:dbl, "error out"=w441:errorcluster)  [unwired: 11 in]
        n157 = Multiply(x=w444, y=1000.0) -> (x*y=→"Photon time (ms)":dbl)
        n158 = call <vilib>:"DAQmx Clear Task.vi"("task in"=w440, "error in"=w441) -> ()  [unwired: 13 in, 1 out]
      }
      frame "WaitObserverResponse" {
        n159 = flat-sequence {
          tunnel: [w479] -> w477
          tunnel: w469 -> [w478]
          tunnel: [w478] -> w470
          tunnel: [w481] -> w476
          tunnel: w477 -> [w481]
          tunnel: [w480] -> w471
          tunnel: w470 -> [w480]
          tunnel: [w512] -> w475
          tunnel: w476 -> [w507]
          tunnel: [w505] -> w468
          tunnel: w471 -> [w505]
          frame #0 {
            n160 = Get Date/Time In Seconds() -> (seconds since 1Jan1904=w479:timestamp)
          }
          frame #1 {
            n161 = while {
              stop <- w485 stop-if-true
              n162 = call "Query Keyboard.vi"("Stop?"=FALSE) -> ("element"=w483:T2)  [unwired: 9 in, 1 out]
              n163 = case shown="Default" w483 {
                tunnel: ["Left" w494 "Right"] -> w484
                frame "D", "F", "S" {
                }
                frame Default {
                  n164 = local read "Observer \nchoice"() -> (w494:string)
                }
                frame "J".."L" {
                }
              }
              "Observer \nchoice" <- w484
              n165 = case shown="Default" w483 {
                tunnel: [0 1 2 3 3 2 1] -> w489
                frame Default {
                }
                frame "S" {
                }
                frame "D" {
                }
                frame "F" {
                }
                frame "J" {
                }
                frame "K" {
                }
                frame "L" {
                }
              }
              n166 = case shown="\"SPACE\"" w483 {
                tunnel: [FALSE TRUE] -> w487
                frame "0", Default {
                }
                frame "SPACE" {
                }
              }
              n167 = local read "Confidence"() -> (w488:i32)
              n168 = Equal To 0?(x=w489) -> (x = 0?=w491:bool)
              n169 = Greater Than 0?(x=w488) -> (x > 0?=w486:bool)
              n170 = And(x=w491, y=w486) -> (x .and. y?=w490:bool)
              n171 = And(x=w487, y=w486) -> (x .and. y?=w485:bool)
              n172 = Select(t=w488, s=w490, f=w489) -> (s? t:f=w492:i32)
              n173 = local write "Confidence"(w492) -> ()
            }
          }
          frame #2 {
            w512 = StateMachineStates_1."CleanUp"  # Next State
            n174 = Get Date/Time In Seconds() -> (seconds since 1Jan1904=w510:timestamp)
            n175 = Subtract(x=w510, y=w507) -> (x-y=w509:dbl)
            n176 = Multiply(x=w509, y=1000.0) -> (x*y=→"Response \ntime (ms)":dbl)
            "Observer Responded" <- TRUE ("Boolean 3")
          }
        }
      }
      frame "CleanUp" {
        n177 = local read "Manual"() -> (w514:bool)
        n178 = local read "Stimulus \nlocation"() -> (w516:string)
        n179 = local read "Observer \nchoice"() -> (w513:string)
        n180 = local read "Blocked trial #"() -> (w515:i32)
        n181 = flat-sequence {
          tunnel: w516 -> [w544]
          tunnel: w513 -> [w543]
          tunnel: w525 -> [w542]
          tunnel: w518 -> [w540]
          tunnel: [w540] -> w517
          frame #0 {
            # "Write data from trial to file."
            n182 = local read "Subject #"() -> (w529:string)
            n183 = Equal?(x=w544, y=w543) -> (x = y?=w546:bool)
            n184 = local read "Trial #"() -> (w533:i32)
            n185 = local read "Counts 2"() -> (w531:u32)
            n186 = local read "Counts 1"() -> (w530:u32)
            n187 = local read "Confidence"() -> (w532:i32)
            n188 = local read "Photon #"() -> (w539:i32)
            n189 = local read "Response \ntime (ms)"() -> (w545:dbl)
            n190 = local read "Photon time (ms)"() -> (w538:dbl)
            n191 = local read "LED Voltage"() -> (w541:dbl)
            n192 = local read "Pump WP"() -> (w534:dbl)
            n193 = call "Prepare data and write to file.vi"("Photon time (ms)"=w538, "String"=w544, "Confidence"=w532, "Photon #"=w539, "Pump WP"=w534, "Observer choice"=w543, "LED Voltage"=w541, "Response \ntime (ms)"=w545, "Path in"=w542, "Boolean"=w546, 10:w533, "Counts in"=w530, "Subject #"=w529, "Counts 1"=w531) -> ()  [unwired: 6 in]
            n194 = feedback #3() -> (w537:dbl[][])  [unwired: 1 in]
            n195 = Build Array(w539, w538, w534) -> (w536:dbl[])
            n196 = Build Array (concatenate)(w536, w537) -> (w535:dbl[][])
            n197 = local write "appended array"(w535) -> ()
            n198 = feedback-in #3(w535) -> ()
          }
        }
        n199 = Array Size(array=w523) -> (size(s)=w522:i32)
        n200 = call "Play sound right wrong.vi"("Audio"="Audio", "String"=w516, "Observer choice"=w513) -> ()  [unwired: 9 in]
        n201 = Equal?(x=w522, y=w515) -> (x = y?=w521:bool)
        n202 = Not(x=w514) -> (.not. x?=w524:bool)
        n203 = And(x=w524, y=w521) -> (x .and. y?=w520:bool)
        n204 = case shown="False" w520 {
          tunnel: [w551 w560] -> w528
          tunnel: w514 -> [_ _]
          frame False {
            # "Display a message and\nswitch to manual mode\nif end of blocked trials\nis reached."
            n205 = case shown="True" "Self-paced" {
              tunnel: [w553 w557] -> w551
              frame False {
                n206 = call "Display Message to User"() -> ("OK"=w552:bool)  [unwired: 10 in, 1 out]
                n207 = case shown="True" w552 {
                  tunnel: [w554 w556] -> w553
                  frame False {
                    w554 = StateMachineStates_1."CleanUp"  # Next State
                  }
                  frame True {
                    w556 = StateMachineStates_1."WaitResearcher"  # Next State
                    n208 = local write "Observer Responded"(FALSE ("Observer Responded")) -> ()
                  }
                }
              }
              frame True {
                w557 = StateMachineStates_1."Setup"  # Next State
                # "Skip \"WaitingResearcher\" mode if trials are self-paced."
                n209 = local write "Observer Responded"(FALSE ("Observer Responded")) -> ()
              }
            }
          }
          frame True {
            n210 = local write "Self-paced"(FALSE ("Self-paced")) -> ()
            n211 = call "Display Message to User2"() -> ("OK"=w561:bool)  [unwired: 10 in, 1 out]
            n212 = case shown="False" w561 {
              tunnel: [w563 w565] -> w560
              frame False {
                w563 = StateMachineStates_1."CleanUp"  # Next State
              }
              frame True {
                w565 = StateMachineStates_1."WaitResearcher"  # Next State
                n213 = local write "Observer Responded"(FALSE ("Observer Responded")) -> ()
              }
            }
            n214 = local write "Manual"(TRUE ("Manual")) -> ()
          }
        }
        n215 = flat-sequence {
          tunnel: [w547] -> w519
          tunnel: w517 -> [w547]
          frame #0 {
            w549 = FALSE ("LC")
            # "Reset indicators"
            n216 = local write "LED Voltage"(0.0 ("LED Voltage")) -> ()
            n217 = local write "Location Set"(w549) -> ()
            n218 = local write "Waiting"(w549) -> ()
            n219 = local write "Stimulus"(w549) -> ()
            n220 = local write "Observer Ready"(w549) -> ()
          }
        }
      }
      frame "Stop" {
        n221 = flat-sequence {
          tunnel: w569 -> [w575]
          tunnel: [w576] -> w568
          tunnel: w568 -> [w578]
          tunnel: [w578] -> w567
          tunnel: [w580] -> w570
          tunnel: w567 -> [w580]
          tunnel: [StateMachineStates_1."Stop" ("Next State")] -> w566
          frame #0 {
            # "Close waveplate session."
            n222 = local read "VISA Handle out"() -> (w574:refnum<visa-resource-name>)
            n223 = call "close.vi"("error in"=w575, "VISA Handle in"=w574) -> ("error out"=w576:errorcluster)  [unwired: 3 in]
          }
          frame #1 {
            w577 = FALSE ("LC")
            # "Reset indicator lights."
            n224 = local write "Stimulus"(w577) -> ()
            n225 = local write "Location Set"(w577) -> ()
            n226 = local write "Observer Responded"(w577) -> ()
            n227 = local write "Waiting"(w577) -> ()
            n228 = local write "Observer Ready"(w577) -> ()
          }
          frame #2 {
          }
        }
      }
    }
  }
